vi "Prueba Servos.vi"() -> ()   [LabVIEW 2021]
uses:
  <vilib>/MakerHub/LINX/Public/Utilities/Open Serial.vi
  <vilib>/MakerHub/LINX/Public/Sensors/Motion/Servo/Servo Open N Channels.vi
  <vilib>/MakerHub/LINX/Public/Sensors/Motion/Servo/Servo Set Pulse Width N Channels.vi
  <vilib>/MakerHub/LINX/Public/Sensors/Motion/Servo/Servo Close N Channels.vi
  <vilib>/MakerHub/LINX/LMH-LINX.lvlib
  <vilib>/MakerHub/LINX/Public/Sensors/Motion/Servo/Servo.lvlib
panel:
  in  "Array":u16[][](array[knob]) scale=500.0..2500.0
  out "Apagado Universal":i16
  out "stop 2":bool
  out "MENSAJE":string
  in  "Puerto":refnum<visa-resource-name>
  out "date/time string":string
  in  "Paro de emergencia":bool
  # "2J&K"
  # "Calibración de servomotores"
  # "Alarma y mensajes"
  # "Fecha y hora"
  # "Configuración de hardware"
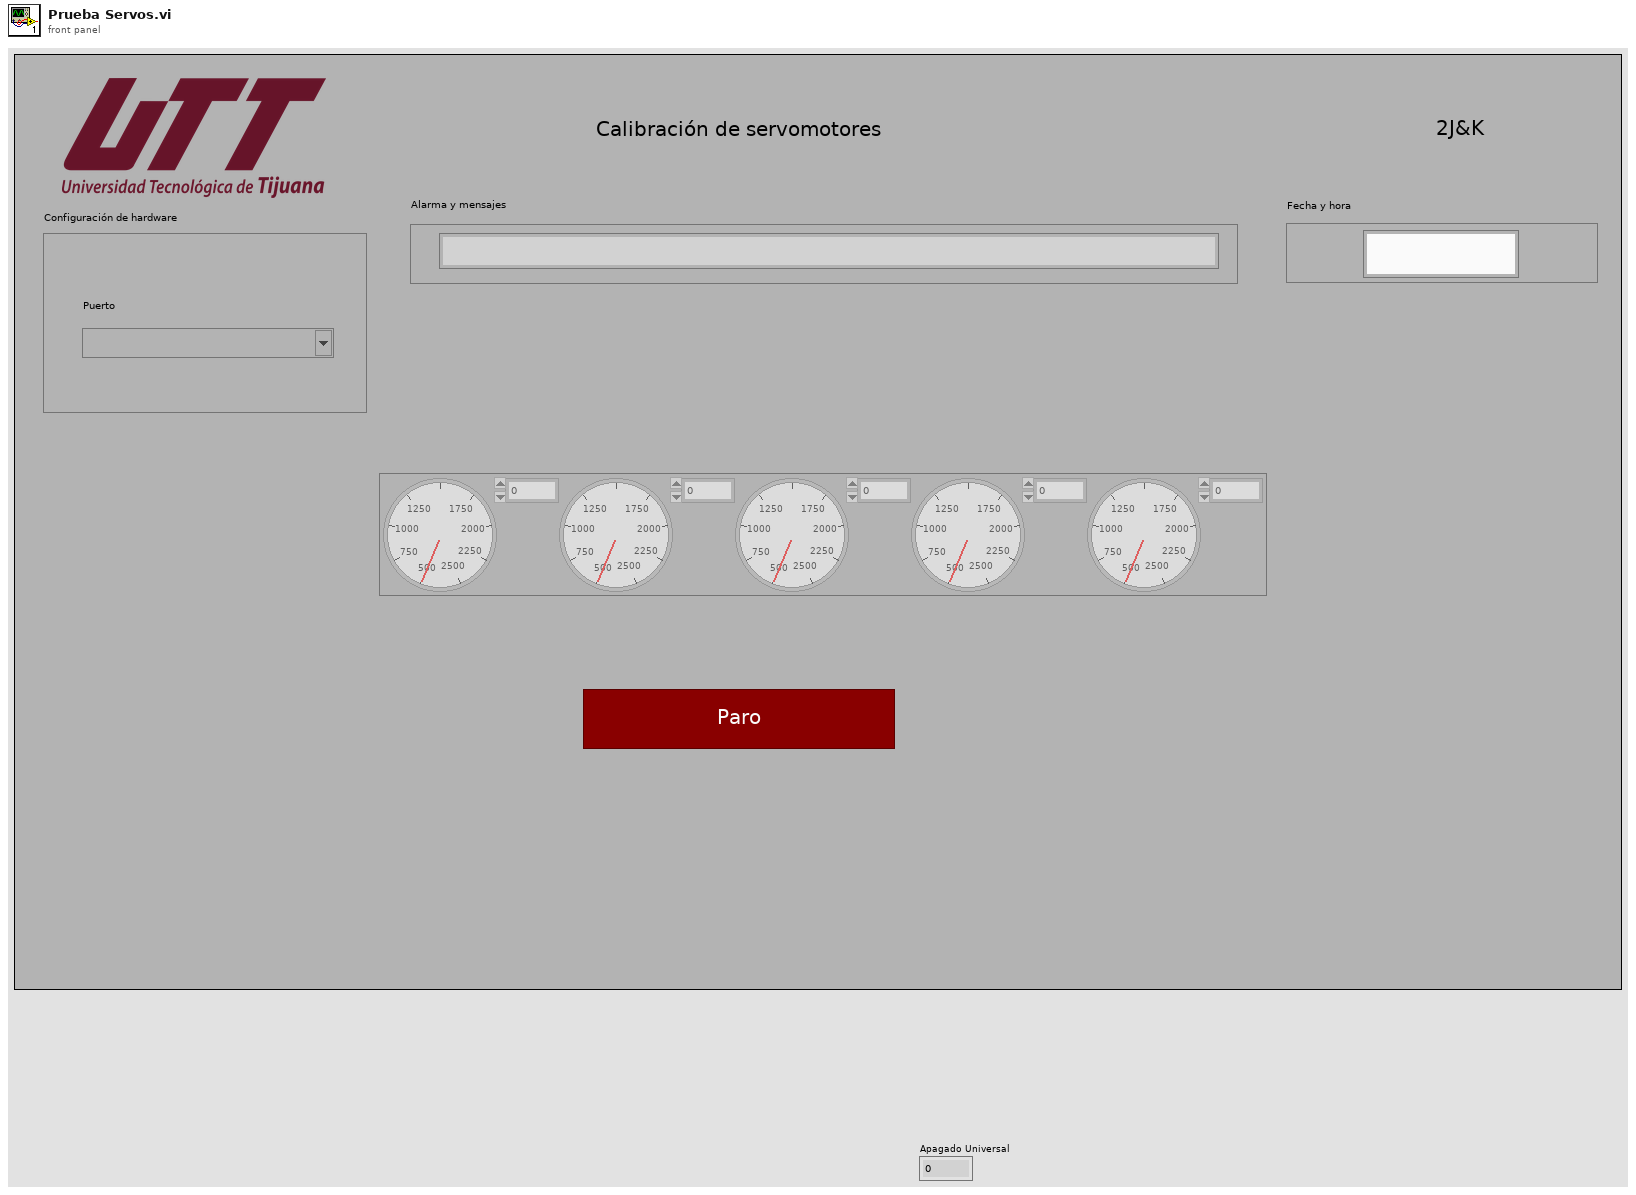
[diagram p1: front panel]
types:
  T1 = typedef "LMH-LINX.lvlib/LINX Ref.ctl" = cluster{"IO":T2, "Interface":T3, "LINX Device Config":T4}
  T2 = typedef "LMH-LINX.lvlib/Platform.ctl" = enum16{"Remote", "Local"}
  T3 = typedef "LMH-LINX.lvlib/Interface.ctl" = enum16{"Serial", "TCP"}
  T4 = typedef "LMH-LINX.lvlib/Device.lvlib/LINX Device Config.ctl" = cluster{"Interface":T3, "COM Port":refnum<visa-resource-name>, "TCP Configuration":T5, "Device Family":u8, "Device ID":u8, "Device Name":string, "TCP Ref":refnum<k5>, "Channels":T6}
  T5 = typedef "LMH-LINX.lvlib/Device.lvlib/TCP Config.ctl" = cluster{"IP Address":string, "Port":u16}
  T6 = typedef "LMH-LINX.lvlib/Channels.ctl" = cluster{"DI":u8[], "DO":u8[], "AI":u8[], "AO":u8[], "PWM":u8[], "QE":u8[], "UART":u8[], "I2C 2":u8[], "SPI":u8[], "CAN":u8[], "Servo":u8[], "AI Ref (V)":dbl, "AI Resolution (Bits)":u8, "AO Ref (V)":dbl, "AO Resolution (Bits)":u8}
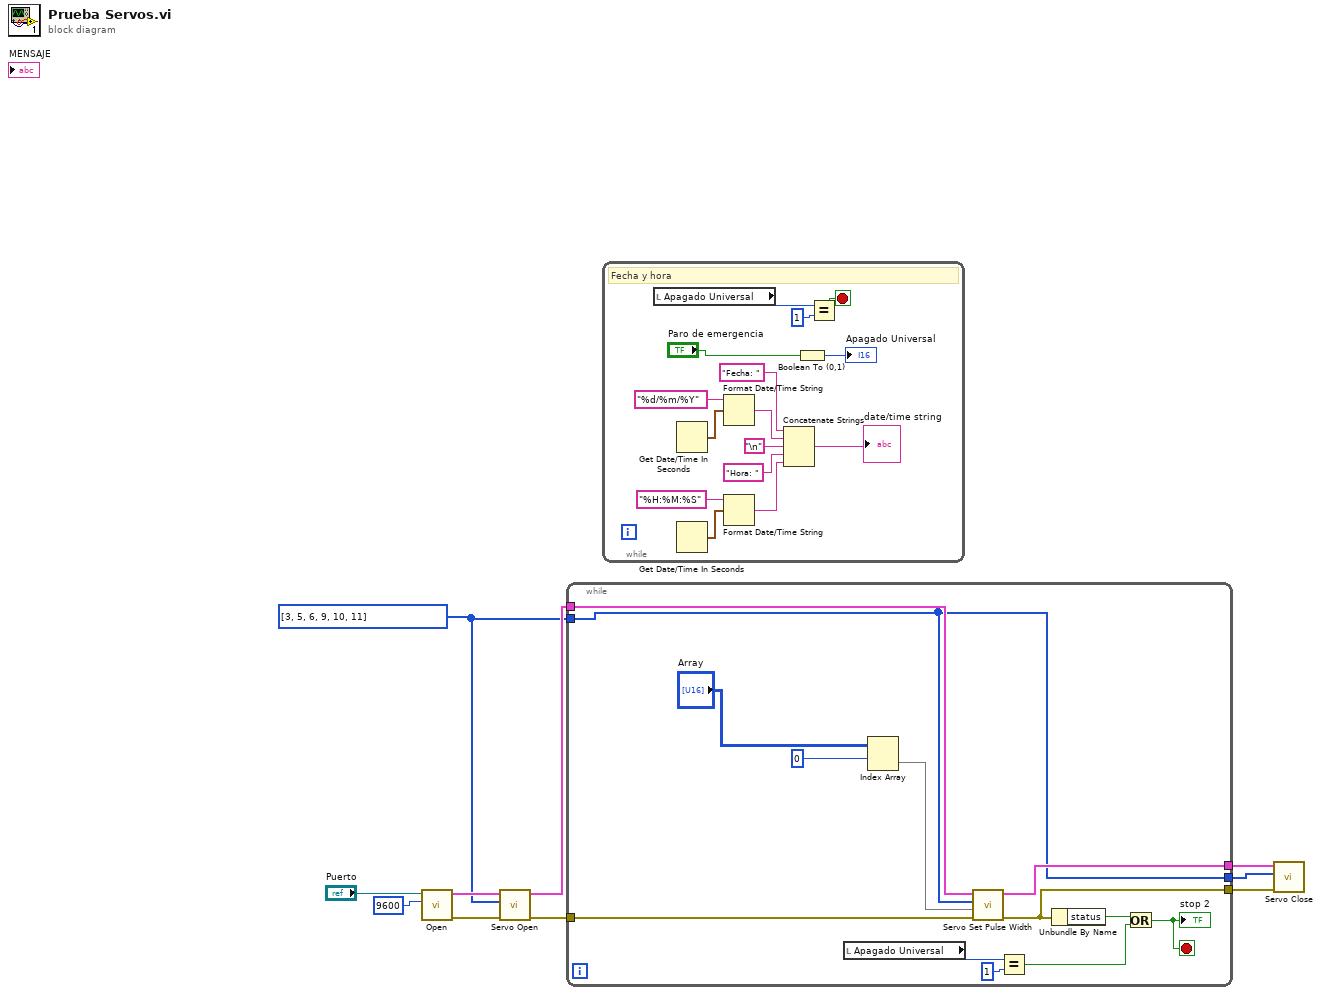
[diagram p0: block diagram]
diagram:
  w2 = u8[] [3, 5, 6, 9, 10, 11]
  n1 = call-poly <vilib>:"Open.vi"("Baud Rate Override"=u32 9600, "Serial Port"="Puerto") -> ("Error Out"=w9:errorcluster, "LINX Resource"=w10:T1)  [unwired: 7 in, 1 out]
  n2 = call-poly <vilib>:"Servo Open.vi"("Error In"=w9, "Servo Channels"=w2, "LINX Resource"=w10) -> ("Error Out"=w5:errorcluster, "LINX Resource"=w6:T1)  [unwired: 7 in]
  n3 = while {
    tunnel: w6 -> [w23]
    tunnel: w5 -> [w22]
    tunnel: [w21] -> w4
    tunnel: [w18] -> w3
    tunnel: w2 -> [w20]
    tunnel: [w20] -> w1
    stop <- w19 stop-if-true
    n4 = local read "Apagado Universal"() -> (w15:i16)
    n5 = Index Array(array="Array", index (row)=0 ("index")) -> (element=w11:u16[])  [unwired: 1 in]
    n6 = call-poly <vilib>:"Servo Set Pulse Width.vi"("Error In"=w22, "Pulse Widths (uS)"=w11, "Servo Channels"=w20, "LINX Resource"=w23) -> ("Error Out"=w18:errorcluster, "LINX Resource"=w21:T1)  [unwired: 6 in]
    n7 = Equal?(x=w15, y=i16 1) -> (x = y?=w14:bool)
    n8 = Unbundle By Name(w18) -> ("status"=w17:bool)
    n9 = Or(x=w17, y=w14) -> (x .or. y?=w19:bool)
    "stop 2" <- w19
  }
  n10 = while {
    stop <- w24 stop-if-true
    # "Fecha y hora"
    n11 = local read "Apagado Universal"() -> (w28:i16)
    n12 = Get Date/Time In Seconds() -> (seconds since 1Jan1904=w35:timestamp)
    n13 = Get Date/Time In Seconds() -> (seconds since 1Jan1904=w36:timestamp)
    n14 = Format Date/Time String(time format string (%c)="%d/%m/%Y", seconds (now)=w35) -> (date/time string=w37:string)  [unwired: 1 in]
    n15 = Format Date/Time String(time format string (%c)="%H:%M:%S", seconds (now)=w36) -> (date/time string=w38:string)  [unwired: 1 in]
    n16 = Concatenate Strings("Fecha: " ("string"), w37, "\n", "Hora: " ("string"), w38) -> (→"date/time string":string)
    n17 = Boolean To (0,1)(Boolean="Paro de emergencia") -> (0, 1=→"Apagado Universal":i16)
    n18 = Equal?(x=w28, y=i16 1) -> (x = y?=w24:bool)
  }
  n19 = call-poly <vilib>:"Servo Close.vi"("Error In"=w3, "Servo Channels"=w1, "LINX Resource"=w4) -> ()  [unwired: 7 in, 2 out]
